vi "OpenCVLib_LoadClassifier.vi"(8 "error in (no error)":errorcluster, 10 "faceCheckerCascadePath":path, 11 "faceCascadePath":path) -> (0 "error out":errorcluster)   [LabVIEW 2019]
uses:
  Binaries/Release/niopencvwrapper.dll
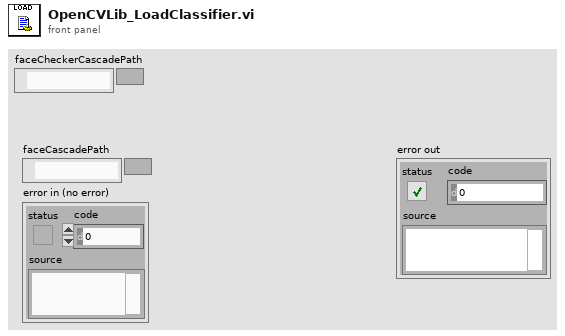
[diagram p1: front panel]
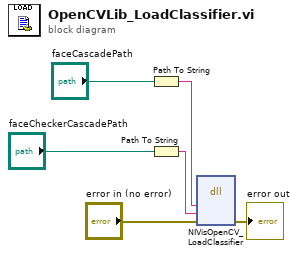
[diagram p0: block diagram]
diagram:
  n1 = Path To String(path="faceCascadePath") -> (string=w5:string)
  n2 = Path To String(path="faceCheckerCascadePath") -> (string=w1:string)
  n3 = dll-call lib="E:/Licenta/trip-validation-system/Binaries/Release/niopencvwrapper.dll" fn="NIVisOpenCV_LoadClassifier"("faceCascadePath"=w5, "faceCheckerCascadePath"=w1, "error"="error in (no error)") -> ("error"=→"error out":errorcluster)  [unwired: 6 in, 2 out]
